vi "Adjust Text to Fit Rectangle.vi"(0 "VI Name":string, 5 "Number of Rows":i32, 7 "Text settings":T1 {"Alignment" items=["left", "center", "right"]}, 9 "Blank Line 1 text?":bool, 11 "Header?":bool) -> (4 "Text out":T4)   [LabVIEW 2024, in "Text-Based VI Icon.lvlib"]
uses:
  <vilib>/LabVIEW Icon API/Set Text Icon/Text-Based VI Icon.lvlib
  <vilib>/LabVIEW Icon API/API_Text.ctl
  <vilib>/LabVIEW Icon API/API_Test Settings.ctl
  <vilib>/LabVIEW Icon API/lv_icon/Controls/Alignment.ctl
  <vilib>/LabVIEW Icon API/API_Text Colors.ctl
  <vilib>/LabVIEW Icon API/LabVIEW Icon API.lvlib
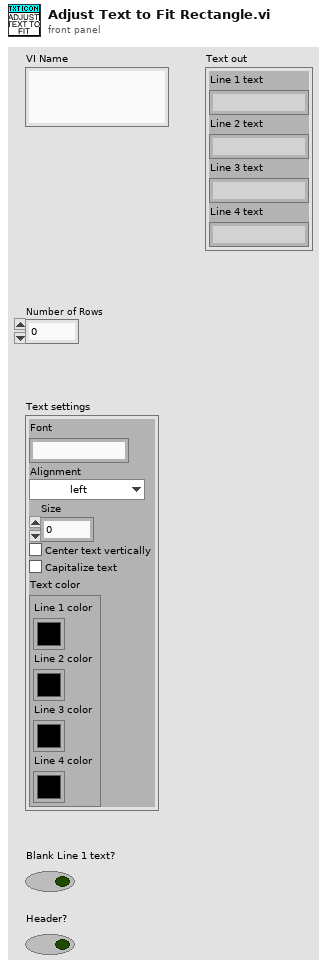
[diagram p1: front panel]
types:
  T1 = typedef "LabVIEW Icon API.lvlib/API_Test Settings.ctl" = cluster{"Font":string, "Alignment":T2, "Size":u8, "Center text":bool, "Capitalize text":bool, "Text color":T3}
  T2 = typedef "Alignment.ctl" = u16
  T3 = typedef "LabVIEW Icon API.lvlib/API_Text Colors.ctl" = cluster{"Line 1 color":u32, "Line 2 color":u32, "Line 3 color":u32, "Line 4 color":u32}
  T4 = typedef "LabVIEW Icon API.lvlib/API_Text.ctl" = cluster{"Line 1 text":string, "Line 2 text":string, "Line 3 text":string, "Line 4 text":string}
  T5 = cluster{"Font Name:":string, "Size":i16, "Strikeout?":bool, "Italic?":bool, "Underline?":bool, "Outline?":bool, "Shadow?":bool, "Bold?":bool}
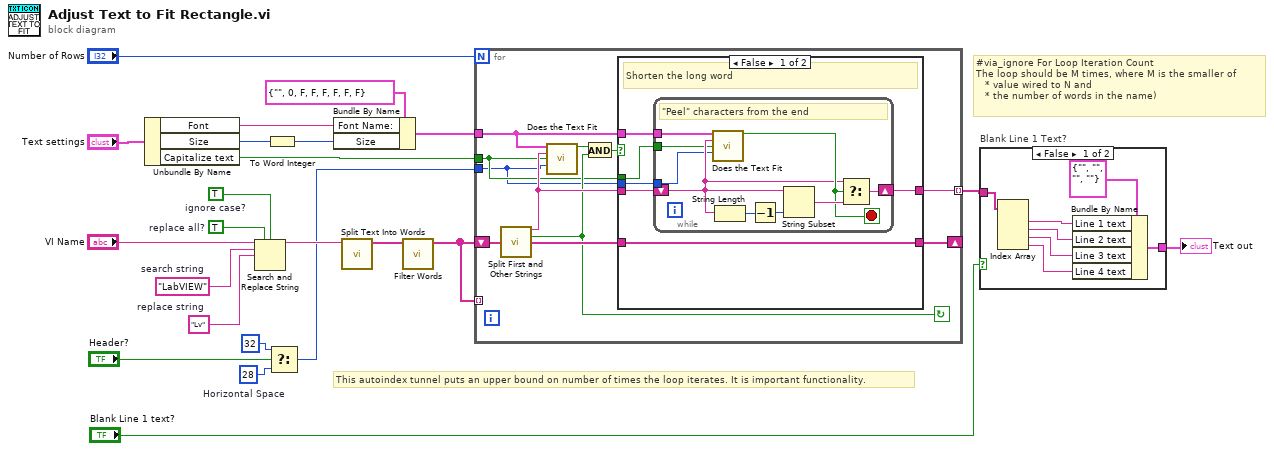
[diagram p0: block diagram]
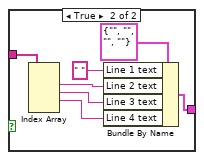
[diagram p2: hidden frame]
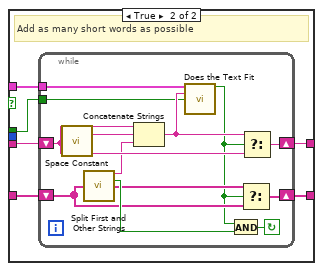
[diagram p3: hidden frame]
diagram:
  w3 = i16 28  # Horizontal Space
  w10 = TRUE  # ignore case?
  w11 = TRUE  # replace all?
  w12 = "Lv"  # replace string
  w13 = "LabVIEW"  # search string
  # "This autoindex tunnel puts an upper bound on number of times the loop iterates. It is important functionality."
  # "#via_ignore For Loop Iteration Count\nThe loop should be M times, where M is the smaller of \n   * value wired to N and \n   * the number of words in the name)"
  n1 = Unbundle By Name("Text settings") -> ("Font"=w20:string, "Size"=w19:u8, "Capitalize text"=w16:bool)
  n2 = Search and Replace String(replace all?=w11, case sensitive?=w10, input string="VI Name", search string=w13, replace string=w12) -> (result string=w8:string)  [unwired: 3 in, 3 out]
  n3 = To Word Integer(number=w19) -> (16bit integer=w17:i16)
  n4 = Select(t=i16 32 ("Horizontal Space"), s="Header?", f=w3) -> (s? t:f=w1:i16)
  n5 = Bundle By Name(cluster=T5 {"Font Name:"="", "Size"=0, "Strikeout?"=FALSE, "Italic?"=FALSE, "Underline?"=FALSE, "Outline?"=FALSE, "Shadow?"=FALSE, "Bold?"=FALSE} ("[user-specified font]"), "Font Name:"=w20, "Size"=w17) -> (w21:T5)
  n6 = call <vilib>:"Split Text Into Words.vi"("VI Name"=w8) -> ("Array"=w15:string[])  [unwired: 10 in]
  n7 = call <vilib>:"Filter Words.vi"("Array in"=w15) -> ("Array out"=w14:string[])  [unwired: 10 in]
  n8 = for {
    N: "Number of Rows" -> [_]
    tunnel: [w26] -> w5 mode=indexing
    tunnel: w21 -> [w33]
    shift-right: [w34] -> _
    shift-left: w14 -> [w30]
    tunnel: w14 -> [_] mode=indexing
    tunnel: w16 -> [w25]
    tunnel: w1 -> [w24]
    stop <- w27 continue-if-true
    n9 = call <vilib>:"Split First and Other Strings.vi"("Strings In"=w30) -> ("First String"=w28:string, "One or More Other Strings"=w27:bool, "Other Strings"=w29:string[])  [unwired: 12 in]
    n10 = call <vilib>:"Does the Text Fit.vi"("user-specified font"=w33, "token string"=w28, "Capitalize Text"=w25, "Horizontal Space"=w24) -> ("Text Fits"=w32:bool)  [unwired: 11 in]
    n11 = And(x=w32, y=w27) -> (x .and. y?=w31:bool)
    n12 = case shown="False" w31 {
      tunnel: w33 -> [w37 w55]
      tunnel: w28 -> [w39 w54]
      tunnel: [w38 w53] -> w26
      tunnel: [w40 w52] -> w34
      tunnel: w29 -> [w40 w51]
      tunnel: w25 -> [w36 w50]
      tunnel: w24 -> [w35 _]
      frame False {
        # "Shorten the long word"
        n13 = while {
          shift-right: [w47] -> w38
          shift-left: w39 -> [w43]
          tunnel: w37 -> [w49]
          tunnel: w36 -> [w42]
          tunnel: w35 -> [w41]
          stop <- w46 stop-if-true
          # "\"Peel\" characters from the end"
          n14 = call <vilib>:"Does the Text Fit.vi"("user-specified font"=w49, "token string"=w43, "Capitalize Text"=w42, "Horizontal Space"=w41) -> ("Text Fits"=w46:bool)  [unwired: 11 in]
          n15 = String Length(string=w43) -> (length=w45:i32)
          n16 = Decrement(x=w45) -> (x-1=w44:i32)
          n17 = String Subset(string=w43, length (rest)=w44) -> (substring=w48:string)  [unwired: 1 in]
          n18 = Select(t=w43, s=w46, f=w48) -> (s? t:f=w47:string)
        }
      }
      frame True {
        # "Add as many short words as possible"
        n19 = while {
          shift-right: [w68] -> w53
          shift-left: w54 -> [w65]
          tunnel: w55 -> [w67]
          shift-right: [w63] -> w52
          shift-left: w51 -> [w60]
          tunnel: w50 -> [w56]
          stop <- w62 continue-if-true
          n20 = call <vilib>:"Space Constant.vi"() -> ("String"=w66:string)
          n21 = call <vilib>:"Split First and Other Strings.vi"("Strings In"=w60) -> ("First String"=w58:string, "One or More Other Strings"=w61:bool, "Other Strings"=w59:string[])  [unwired: 12 in]
          n22 = Concatenate Strings(w65, w66, w58) -> (w64:string)
          n23 = call <vilib>:"Does the Text Fit.vi"("user-specified font"=w67, "token string"=w64, "Capitalize Text"=w56) -> ("Text Fits"=w57:bool)  [unwired: 12 in]
          n24 = And(x=w57, y=w61) -> (x .and. y?=w62:bool)
          n25 = Select(t=w59, s=w57, f=w60) -> (s? t:f=w63:string[])
          n26 = Select(t=w64, s=w57, f=w65) -> (s? t:f=w68:string)
        }
      }
    }
  }
  n27 = case "Blank Line 1 Text?" shown="False" "Blank Line 1 text?" {
    tunnel: [w75 w76] -> w7
    tunnel: w5 -> [w70 w78]
    frame False {
      n28 = Index Array(array=w70) -> (element #1=w71:string, element #2=w72:string, element #3=w73:string, element #4=w74:string)  [unwired: 4 in]
      n29 = Bundle By Name(cluster=T4 {"Line 1 text"="", "Line 2 text"="", "Line 3 text"="", "Line 4 text"=""} ("Text out"), "Line 1 text"=w71, "Line 2 text"=w72, "Line 3 text"=w73, "Line 4 text"=w74) -> (w75:T4)
    }
    frame True {
      n30 = Index Array(array=w78) -> (element #1=w80:string, element #2=w81:string, element #3=w82:string)  [unwired: 4 in, 1 out]
      n31 = Bundle By Name(cluster=T4 {"Line 1 text"="", "Line 2 text"="", "Line 3 text"="", "Line 4 text"=""} ("Text out"), "Line 1 text"=" ", "Line 2 text"=w80, "Line 3 text"=w81, "Line 4 text"=w82) -> (w76:T4)
    }
  }
  "Text out" <- w7
